vi "svc_Integral Ydx.vi"(6 "state in":cluster{"x":dbl, "y":dbl, "integral":dbl}, 7 "reset":bool, 11 "XY":cluster{"X":dbl[], "Y":dbl[]}(graph)) -> (3 "Integral":cluster{"X":dbl[], "Y":dbl[]}(graph), 4 "state out":cluster{"x":dbl, "y":dbl, "integral":dbl})   [LabVIEW 2017]
doc: "computes the integral of Y with respect to X\n\ncareful, this VI does not perform error checking and can return negative integral if positive function is integrated from right to left (this might even be useful if you are trying to find the area enclosed by a set of points)"
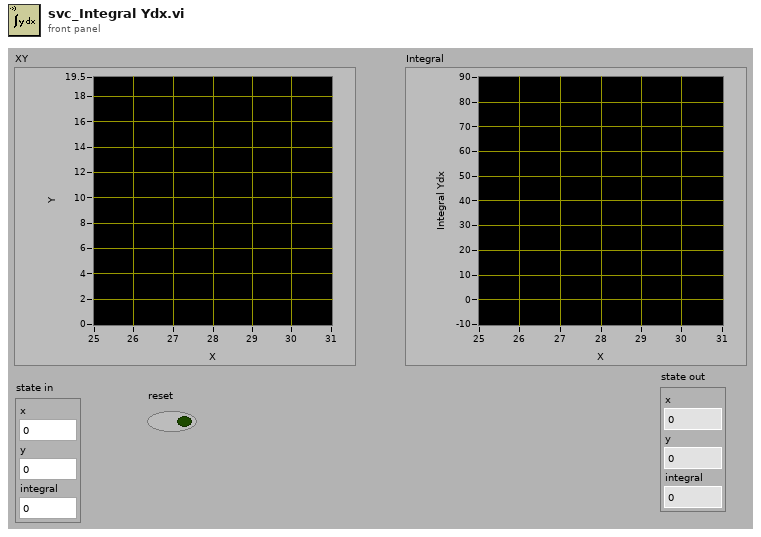
[diagram p1: front panel]
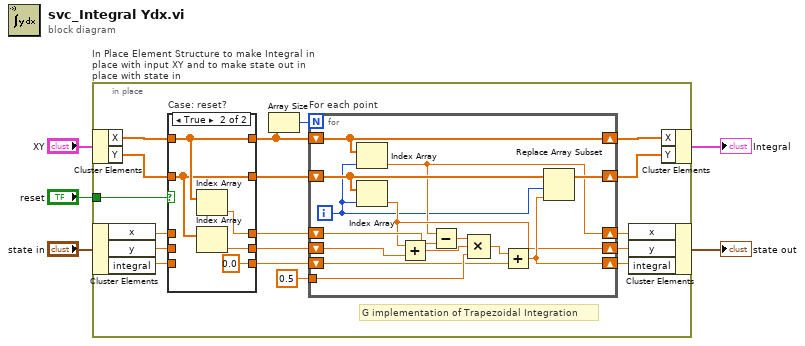
[diagram p0: block diagram]
diagram:
  n1 = in-place "In Place Element Structure to make Integral in place with input XY and to make state out in place with state in" {
    in-place-border: "reset" -> [w21]
    # "G implementation of Trapezoidal Integration"
    n2 = in-place-cluster #1("XY") -> ("X"=w20:dbl[], "Y"=w19:dbl[])
    n3 = in-place-cluster #2("state in") -> ("x"=w18:dbl, "y"=w17:dbl, "integral"=w16:dbl)
    n4 = case "Case: reset?" shown="True" w21 {
      tunnel: w20 -> [w28 w33]
      tunnel: [w28 w33] -> w6
      tunnel: w19 -> [w27 w32]
      tunnel: [w27 w32] -> w9
      tunnel: w18 -> [w26 _]
      tunnel: [w26 w31] -> w14
      tunnel: w17 -> [w25 _]
      tunnel: [w25 w30] -> w13
      tunnel: w16 -> [w24 _]
      tunnel: [w24 0.0 ("integral")] -> w15
      frame False {
      }
      frame True {
        n5 = Index Array(array=w33) -> (element=w31:dbl)  [unwired: 1 in]
        n6 = Index Array(array=w32) -> (element=w30:dbl)  [unwired: 1 in]
      }
    }
    n7 = Array Size(array=w6) -> (size(s)=w7:i32)
    n8 = for "For each point" {
      N: w7 -> [_]
      shift-right: [w46] -> w22
      shift-left: w15 -> [w40]
      shift-right: [w47] -> w23
      shift-left: w9 -> [w45]
      shift-right: [w35] -> w11
      shift-left: w14 -> [w44]
      shift-right: [w37] -> w10
      shift-left: w13 -> [w43]
      tunnel: 0.5 ("y") -> [w41]
      shift-right: [w36] -> w8
      shift-left: w6 -> [w36]
      i -> [w34]
      n9 = Index Array(array=w36, index=w34) -> (element=w35:dbl)
      n10 = Index Array(array=w45, index=w34) -> (element=w37:dbl)
      n11 = Add(x=w37, y=w43) -> (x+y=w42:dbl)
      n12 = Subtract(x=w35, y=w44) -> (x-y=w38:dbl)
      n13 = Compound Arithmetic op=MULTIPLY(w38, w42, w41) -> (w39:dbl)
      n14 = Add(x=w39, y=w40) -> (x+y=w46:dbl)
      n15 = Replace Array Subset(array=w45, new element=w46, index=w34) -> (w47:dbl[])
    }
    n16 = in-place-cluster #2("x"=w11, "y"=w10, "integral"=w22) -> (→"state out":cluster{"x":dbl, "y":dbl, "integral":dbl})
    n17 = in-place-cluster #1("X"=w8, "Y"=w23) -> (→"Integral":cluster{"X":dbl[], "Y":dbl[]})
  }
